vi "Experiment Initialization.vi"(0 "Header Comments":string="This is a C(T) experiment being done in Physics 350.\r\nIt records the decay response of an RC circuit where the capacitance is a strong function of temperature.", 5 "Temperature Control Parameters":T3={"Start Temp"=40.0, "Temp Step"=10.0, "End Temp"=60.0} {"End Temp" format="%.2f"; "Temp Step" format="%.2f"; "Start Temp" format="%.2f"}, 9 "Timing Control Parameters":T2={"N cycles for averaging"=30, "N points per measurement"=1000, "Measurment time interval"=1e-05} {"Measurment time interval" format="%.2e"}, 11 "error in (no error)":errorcluster) -> (2 "Go Forward":bool, 3 "Auto Launch Data Viewer at End":bool=TRUE, 4 "data file path out":path, 6 "Temp Array":dbl[](array[numeric])=[40.0, 50.0, 60.0] format="%.2f", 8 "Timing Control Parameters out":T1={"N cycles for averaging"=100, "N points per measurment"=1000, "Measurment time interval"=1e-05} {"Measurment time interval" format="%.2e"}, 15 "error out":errorcluster)   [LabVIEW 2016]
doc: "This vi starts the C(T) expermental sequence. It creates the control parameters necessary for the rest of the experimental sequence. It allows for the option of loading the parameters from a pre-built template text file as well.\n\nPaul K Dixon\nPhysics 350\nCSUSB Physics"
uses:
  globals/C(T) global variables.vi
panel:
  in  "reload parameters":bool
  in  "default init data file name":string="P350 C(T) experimental data file"
  in  "exit":bool
  in  "go forward":bool
  out "File Header":string="This is a C(T) experiment being done in Physics 350.\r\nIt records the decay response of an RC circuit where the capacitance is a strong function of temperature.\r\n\r\n2/13/2004\r\n11:00 AM\r\n\r\nStart temp = 40.0\r\nTemp step = 10.0\r\nEnd temp = 60.0\r\nNum temps = 3\r\nNum avg cycles = 100\r\nNum points per meas = 1000\r\nMeas time interval = 1.00E-5\r\n\r\nDDD\r\n\r\n"
  out "N temps":i32=3
  in  "Auto Launch Data Viewer at End":bool=TRUE
  # "P350 C(T) Experimental Initialization"
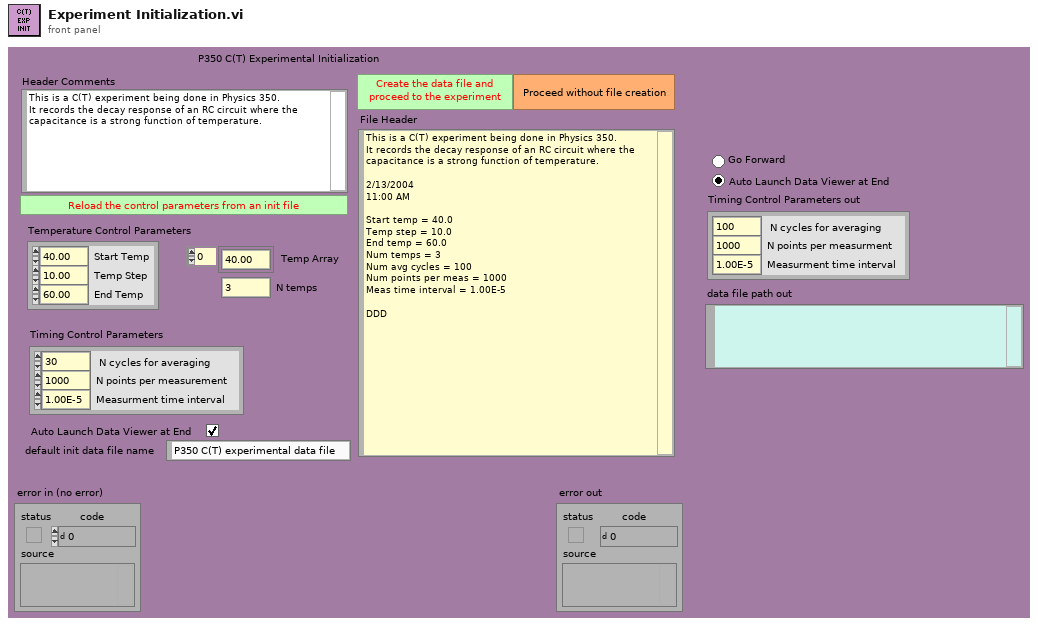
[diagram p1: front panel]
types:
  T1 = cluster{"N cycles for averaging":i32, "N points per measurment":i32, "Measurment time interval":dbl}
  T2 = cluster{"N cycles for averaging":i32, "N points per measurement":i32, "Measurment time interval":dbl}
  T3 = cluster{"Start Temp":dbl, "Temp Step":dbl, "End Temp":dbl}
  T4 = cluster{"Starting Value":dbl, "Step size":dbl, "Ending Value":dbl}
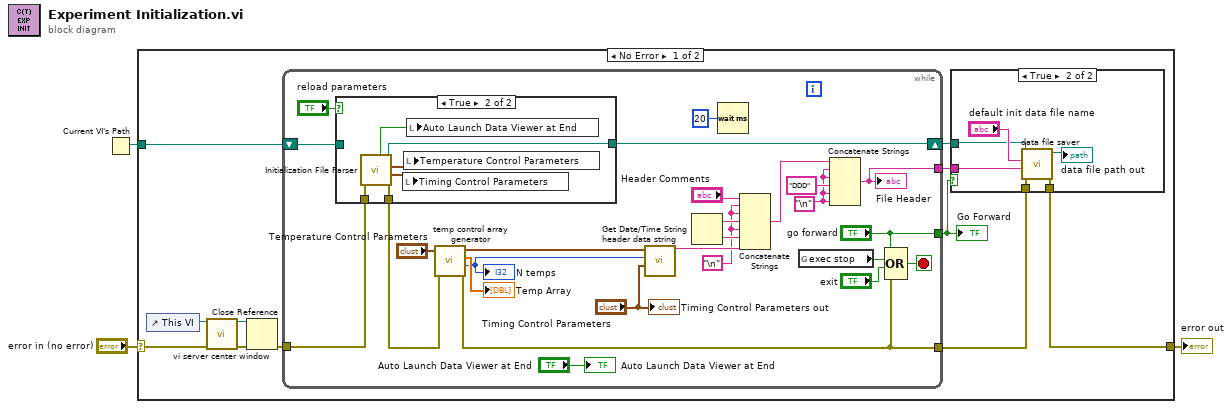
[diagram p0: block diagram]
diagram:
  n1 = Current VI's Path() -> (path=w1:path)
  n2 = case shown="No Error" "error in (no error)" {
    selector: "error in (no error)" -> [w7 w56]
    tunnel: [w11 w56] -> w3
    tunnel: w1 -> [w10 _]
    frame No Error {
      n3 = control-ref of="This VI"() -> (w8:refnum<vi>)
      n4 = call "vi server center window.vi"("VI ref in"=w8, "error in"=w7) -> ("VI ref out"=w4:refnum<vi>, "error out"=w6:errorcluster)  [unwired: 12 out]
      n5 = Close Reference(reference=w4, error in (no error)=w6) -> (error out=w5:errorcluster)
      n6 = while {
        shift-left: w10 -> [w22]
        shift-right: [w21] -> w9
        tunnel: ["go forward"] -> w13
        tunnel: [w40] -> w14
        tunnel: w5 -> [w16]
        tunnel: [w15] -> w12
        stop <- w19 stop-if-true
        w35 = "\n"
        w32 = "\n"
        n7 = case shown="True" "reload parameters" {
          tunnel: [w42 w46] -> w24
          tunnel: [w41 w45] -> w21
          tunnel: w16 -> [w42 w43]
          tunnel: w22 -> [w41 _]
          frame False {
          }
          frame True {
            n8 = call "Initialization File Parser.vi"("error in (no error)"=w43) -> ("error out"=w46:errorcluster, "Timing Control Parameters"=w47:T2, "Temperature Control Parameters"=w48:T3, "file path used"=w45:path, "Auto Launch Data Viewer at End"=w44:bool)  [unwired: 1 in, 5 out]
            n9 = local write "Timing Control Parameters"(w47) -> ()
            n10 = local write "Temperature Control Parameters"(w48) -> ()
            n11 = local write "Auto Launch Data Viewer at End"(w44) -> ()
          }
        }
        n12 = call "temp control array generator.vi"("error in (no error)"=w24, "T control in"="Temperature Control Parameters") -> ("error out"=w15:errorcluster, "N temps"=w28:i32, "Temp Values"=→"Temp Array":dbl[], "T control out"=w29:T4)  [unwired: 3 in, 3 out]
        "N temps" <- w28
        n13 = call "header data string.vi"("Timing Control Parameters"="Timing Control Parameters", "N temps"=w28, "Temperature Control Parameters"=w29) -> ("Concatenated String"=w39:string)  [unwired: 5 in, 3 out]
        n14 = Get Date/Time String() -> (date string=w38:string, time string=w37:string)  [unwired: 3 out]
        n15 = Wait (ms)(milliseconds to wait=u32 20) -> ()  [unwired: 1 out]
        n16 = Concatenate Strings("Header Comments", w32, w32, w38, w32, w37, w39) -> (w33:string)
        n17 = global read "C(T) global variables.vi" "exec stop"() -> (w18:bool)
        n18 = Concatenate Strings(w33, w35, w35, "DDD", w35, w35) -> (w40:string)
        "File Header" <- w40
        n19 = Compound Arithmetic op=OR("go forward", w18, "exit", w15) -> (w19:bool)
        "Auto Launch Data Viewer at End" <- "Auto Launch Data Viewer at End"
        "Timing Control Parameters out" <- "Timing Control Parameters"
      }
      "Go Forward" <- w13
      n20 = case shown="True" w13 {
        tunnel: w14 -> [_ w55]
        tunnel: w9 -> [_ w52]
        tunnel: w12 -> [w49 w51]
        tunnel: [w49 w50] -> w11
        frame False {
        }
        frame True {
          n21 = call "data file saver.vi"("error in (no error)"=w51, "Header String"=w55, "default data file name"="default init data file name", "reference file path in"=w52) -> ("error out"=w50:errorcluster, "data file path out"=→"data file path out":path)  [unwired: 6 out]
        }
      }
    }
    frame Error {
    }
  }
  "error out" <- w3
